vi "Read N Circles Radius.vi"(8 "Error In":errorcluster, 11 "Leap Handle":T2) -> (0 "Error Out":errorcluster, 1 "Circle Statuses":T1[](array[typedef]), 2 "All Circle Progress":dbl[](array[numeric]), 3 "Leap Handle":T2)   [LabVIEW 2011, in "LMH-Leap.lvlib"]
doc: "Read N circle gestures radiuses."
uses:
  LMH-Leap.lvlib
  Private/Type Defs/Leap Handle.ctl
  C:/github/makerhub/Leap/LabVIEW/vi.lib/MakerHub/Leap/Private/Libs/LeapCSharp.NET3.5.dll
  Private/Libs/LeapCSharp.NET3.5.dll
  Private/Type Defs/Gesture State.ctl
  Read N Circles.vi
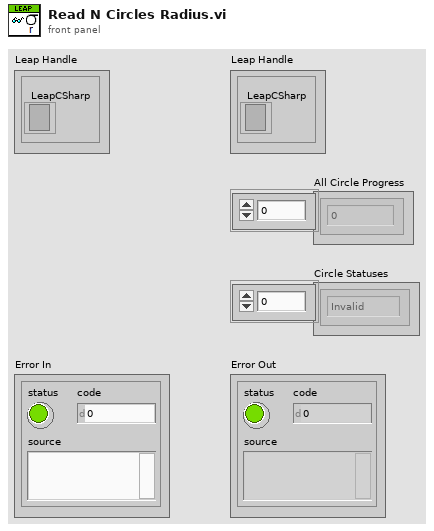
[diagram p1: front panel]
types:
  T1 = typedef "LMH-Leap.lvlib/Gesture State.ctl" = enum16{"Invalid", "Start", "Update", "Stop"}
  T2 = typedef "LMH-Leap.lvlib/Leap Handle.ctl" = cluster{"LeapCSharp":refnum<k24>}
  T3 = typedef "LMH-Leap.lvlib/Gesture Circle.ctl" = cluster{"Common":T4, "Center":T6, "Normal":T6, "Progress":dbl, "Radius":dbl}
  T4 = typedef "LMH-Leap.lvlib/Gesture Common.ctl" = cluster{"ID":dbl, "Duration (S)":dbl, "Gesture Type":T5, "Gesture State":T1}
  T5 = typedef "LMH-Leap.lvlib/Gesture Type.ctl" = enum16{"Invalid", "Swipe", "Circle", "Screen Tap", "Key Tap"}
  T6 = typedef "LMH-Leap.lvlib/Vector.ctl" = cluster{"Pitch":sgl, "Yaw":sgl, "Roll":sgl, "Magnitude":sgl, "XYZ":sgl[]}
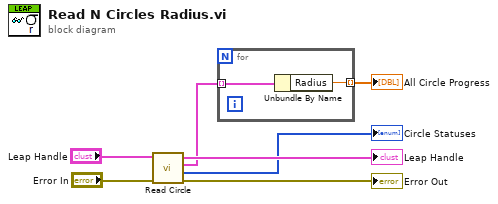
[diagram p0: block diagram]
diagram:
  n1 = call-poly "Read Circle.vi"("Error In"="Error In", "Leap Handle"="Leap Handle") -> ("Error Out"=→"Error Out":errorcluster, "Circle Statuses"=→"Circle Statuses":T1[], "All Circles Data"=w3:T3[], "Leap Handle"=→"Leap Handle":T2)  [unwired: 6 in]
  n2 = for {
    tunnel: [w9] -> w2 mode=indexing
    tunnel: w3 -> [w8] mode=indexing
    n3 = Unbundle By Name(w8) -> ("Radius"=w9:dbl)
  }
  "All Circle Progress" <- w2
